vi "OW Reset.vi"(10 "ChannelMask":u32, 11 "DevHandle":i32) -> (3 "function return":i32)   [LabVIEW 2010, in "usb2ow.lvlib"]
doc: "int WINAPI OW_Reset(int DevHandle, unsigned int ChannelMask);"
uses:
  usb2ow.lvlib
  USB2XXX/trunk/USB2XXX/USB2XXX/vs2010/Release/USB2XXX.dll
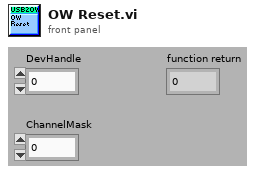
[diagram p1: front panel]
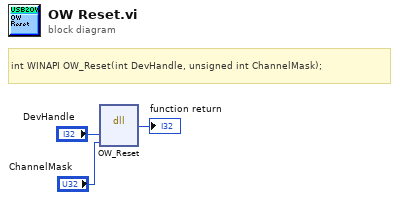
[diagram p0: block diagram]
diagram:
  # "int WINAPI OW_Reset(int DevHandle, unsigned int ChannelMask);"
  n1 = dll-call lib="E:/OtherWork/STM32/USB2XXX/trunk/USB2XXX/USB2XXX/vs2010/Release/USB2XXX.*" fn="OW_Reset"("DevHandle"="DevHandle", "ChannelMask"="ChannelMask") -> (→"function return":i32)  [unwired: 5 in, 2 out]
